vi "Get norm to um scaling .vi"(8 "error in (no error)":errorcluster, 11 "Current Objective":string) -> (0 "error out":errorcluster, 2 "X_norm to um_scaling":dbl, 3 "Z_norm to um_scaling":dbl)   [LabVIEW 2017]
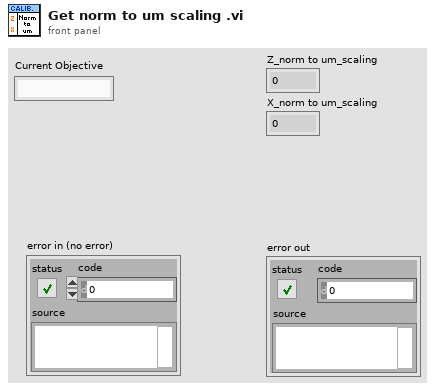
[diagram p1: front panel]
types:
  T1 = enum16{"Initialise", "Load from file", "Save to file", "Read", "Write"}
  T2 = typedef "Calibration config.ctl" = cluster{"Current Objective":string, "Objective Settings":T3[], "PreChirper Values Preset ?":bool, "PreChirper Settings":T4[], "PreChirper Constants":T5}
  T3 = typedef "Objective Config.ctl" = cluster{"Name":string, "Sum X":dbl, "Sum Y":dbl, "Diff X":dbl, "Diff Y":dbl, "Distortion Correction":dbl, "Z_norm to um_scaling":dbl, "X_norm to um_scaling":dbl, "Calibrated Wavelength":dbl}
  T4 = typedef "Prechirper Cal Config.ctl" = cluster{"Wavelength":i32, "Prism 1":i32, "Prism 2":i32}
  T5 = typedef "PreChirper constants.ctl" = cluster{"a 1":i32, "b 1":i32, "c 1":i32, "a 2":i32, "b 2":i32, "c 2":i32, "lmin":i32, "lmax":i32}
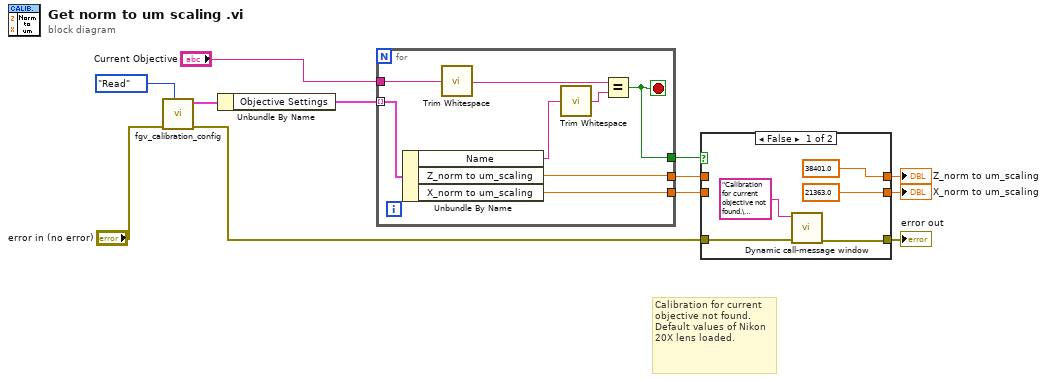
[diagram p0: block diagram]
diagram:
  # "Calibration for current objective not found.\nDefault values of Nikon 20X lens loaded."
  n1 = call "fgv_calibration_config.vi"("Cal config ops"=T1."Read", "error in (no error)"="error in (no error)") -> ("error out"=w3:errorcluster, "Config cluster OUT"=w11:T2)  [unwired: 8 in]
  n2 = Unbundle By Name(w11) -> ("Objective Settings"=w10:T3[])
  n3 = for {
    tunnel: "Current Objective" -> [w19]
    tunnel: w10 -> [w20] mode=indexing
    tunnel: [w15] -> w8
    tunnel: [w14] -> w6
    tunnel: [w13] -> w9
    stop <- w13 stop-if-true
    n4 = Unbundle By Name(w20) -> ("Name"=w18:string, "Z_norm to um_scaling"=w15:dbl, "X_norm to um_scaling"=w14:dbl)
    n5 = call <vilib>:"Trim Whitespace.vi"("string"=w19) -> ("trimmed string"=w16:string)  [unwired: 1 in]
    n6 = call <vilib>:"Trim Whitespace.vi"("string"=w18) -> ("trimmed string"=w17:string)  [unwired: 1 in]
    n7 = Equal?(x=w16, y=w17) -> (x = y?=w13:bool)
  }
  n8 = case shown="False" w9 {
    tunnel: w8 -> [_ w28]
    tunnel: [38401.0 ("Z_norm to um_scaling") w28] -> w7
    tunnel: w6 -> [_ w27]
    tunnel: [21363.0 ("X_norm to um_scaling") w27] -> w5
    tunnel: w3 -> [w23 w26]
    tunnel: [w22 w26] -> w2
    frame False {
      n9 = call "Dynamic call-message window.vi"("error in (no error)"=w23, "Message"="Calibration for current objective not found.\nDefault values of Nikon 20X lens loaded. ") -> ("error out"=w22:errorcluster)  [unwired: 9 in]
    }
    frame True {
    }
  }
  "Z_norm to um_scaling" <- w7
  "X_norm to um_scaling" <- w5
  "error out" <- w2
